vi "DFD NStage MRate Filtering (Array).vi"(6 "zero phase? (T)":bool=TRUE, 7 "init? (F)":bool, 8 "error in (no error)":errorcluster, 10 "multirate filters":T1[](array[typedef]) {"mMRate_SumWl" min=1 max=32 step=1; "mMRate_InputIwl" min=1 max=32 step=1; "mMRate_GainWl" min=1 max=32 step=1; "mMRate_OutputWl" min=1 max=32 step=1; "mMRate_InputWl" min=1 max=32 step=1; "mMRate_CoefWl" min=1 max=32 step=1; "mMRate_Mode" items=["Default"=-1, "No Rate Change"=0, "Interpolation"=1, "Decimation"=2, "Interpolated"=3, "Rational"=4]}, 11 "signal in":dbl[](array[numeric])) -> (0 "error out":errorcluster, 3 "signal out":dbl[](array[numeric]))   [LabVIEW 2017, in "NI_DigFilterLicensed.lvlib"]
doc: "Filters a signal continuously with a multistage multirate filter. Wire data to the <B>signal in</B> input to determine the polymorphic instance to use or manually select the instance."
uses:
  <vilib>/addons/Digital Filter Design/NI_DigFilterLicensed.lvlib
  <vilib>/addons/Digital Filter Design/_Objects.llb/DFD Multirate Filter Obj.ctl
  <vilib>/addons/Digital Filter Design/_Objects.llb/DFD Multirate Mode.ctl
  <vilib>/addons/Digital Filter Design/_Objects.llb/DFD Coef Norm Type.ctl
  <vilib>/addons/Digital Filter Design/_Objects.llb/DFD Round-off Mode.ctl
  <vilib>/addons/Digital Filter Design/_Objects.llb/DFD FXP MRate Multiply Mode.ctl
  <vilib>/addons/Digital Filter Design/NI_DigFilter_Process.lvlib
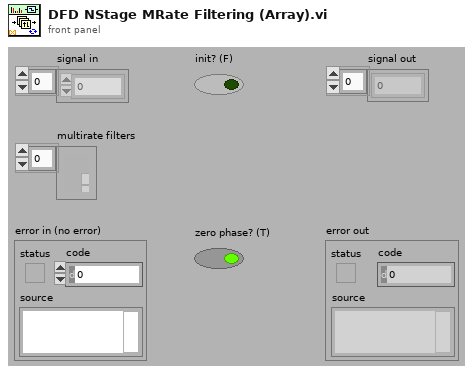
[diagram p1: front panel]
types:
  T1 = typedef "NI_DigFilterLicensed.lvlib/DFD Multirate Filter Obj.ctl" = cluster{"mMRate_Structure":enum16{"CIC", "FIR", "IIR", "Lattice"}, "mMRate_Mode":T2, "mMRate_Factor":i32, "mMRate_FIRParams":cluster{"mMRate_FIR_H":dbl[], "mMRate_FIR_IsNyquist?":bool, "mMRate_FIR_IsSymmetric?":bool}, "mMRate_CICParams":cluster{"mMRate_CIC_#Stage":i32, "mMRate_CIC_Lag":i32, "mMRate_CIC_Type":enum16{"Lowpass", "Highpass"}}, "mMRate_Order":i32, "mMRate_Version":string, "mMRate_Comments":string, "mMRate_RationalFactor":cluster{"mMRate_L":i32, "mMRate_M":i32}, "mMRate_Fs":dbl, "mMRate_Quantized?":bool, "mMRate_QFilterGain":dbl, "mMRate_CoefWl":i16, "mMRate_Scaling":cluster{"mMRate_ScaleByPowerOf2?":bool, "mMRate_ScaleType":T3}, "mMRate_InputWl":i16, "mMRate_OutputWl":i16, "mMRate_OutputMode":T4, "mMRate_MultMode":T5, "mMRate_BitPruning":bool, "mMRate_GainWl":i16, "mMRate_OutputFwl":i16, "mMRate_SumIwl":i16, "mMRate_InputIwl ":i16, "mMRate_SumWl":i16, "mMRate_CoefIwl":i16}
  T2 = typedef "NI_DigFilterLicensed.lvlib/DFD Multirate Mode.ctl" = i16
  T3 = typedef "NI_DigFilterLicensed.lvlib/DFD Coef Norm Type.ctl" = enum16{"No Norm", "Time Domain 1-Norm", "Time Domain 2-Norm", "Time Domain Inf-Norm"}
  T4 = typedef "NI_DigFilterLicensed.lvlib/DFD Round-off Mode.ctl" = enum16{"Nearest", "Truncation"}
  T5 = typedef "NI_DigFilterLicensed.lvlib/DFD FXP MRate Multiply Mode.ctl" = enum16{"Truncated", "Full"}
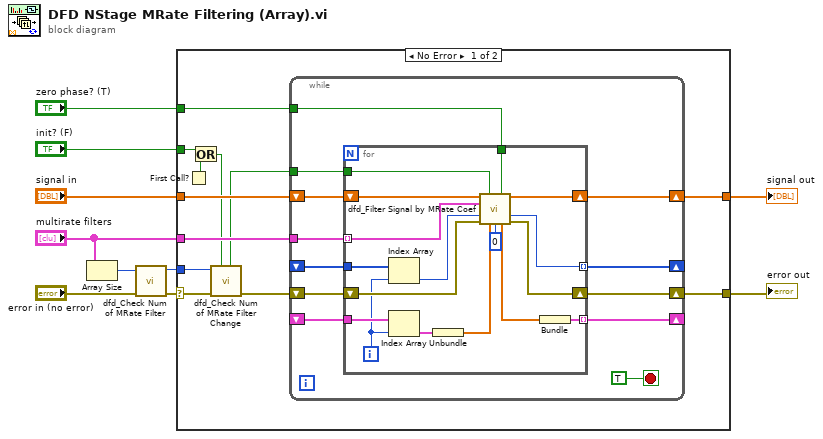
[diagram p0: block diagram]
diagram:
  n1 = Array Size(array="multirate filters") -> (size(s)=w3:i32)
  n2 = call <vilib>:"dfd_Check Num of MRate Filter.vi"("error in (no error)"="error in (no error)", "#MRate in"=w3) -> ("error out"=w4:errorcluster, "#MRate out"=w1:i32)  [unwired: 8 out]
  n3 = case shown="No Error" w4 {
    selector: w4 -> [w15 w52]
    tunnel: [w22 w52] -> w10
    tunnel: "multirate filters" -> [w16 _]
    tunnel: "signal in" -> [w17 _]
    tunnel: [w20 _] -> w8
    tunnel: "zero phase? (T)" -> [w21 _]
    tunnel: "init? (F)" -> [w18 _]
    tunnel: w1 -> [w11 _]
    frame No Error {
      n4 = First Call?() -> (First Call?: T/F=w19:bool)
      n5 = Or(x=w18, y=w19) -> (x .or. y?=w13:bool)
      n6 = call <vilib>:"dfd_Check Num of MRate Filter Change.vi"("init in"=w13, "error in (no error)"=w15, "#MRate in"=w11) -> ("error out"=w14:errorcluster, "init out"=w12:bool)  [unwired: 7 out]
      n7 = while {
        tunnel: w16 -> [w34]
        shift-right: [w32] -> _
        shift-left: _ -> [w26]
        tunnel: w12 -> [w27]
        shift-right: [w30] -> _
        shift-left: _ -> [w24]
        tunnel: w21 -> [w23]
        shift-right: [w25] -> w22
        shift-left: w14 -> [w31]
        shift-right: [w28] -> w20
        shift-left: w17 -> [w29]
        stop <- TRUE stop-if-true
        n8 = for {
          tunnel: w34 -> [w47] mode=indexing
          tunnel: [w51] -> w32 mode=indexing
          tunnel: w26 -> [w50]
          tunnel: [w46] -> w30 mode=indexing
          tunnel: w27 -> [w35]
          tunnel: w23 -> [w45]
          shift-right: [w44] -> w28
          shift-left: w29 -> [w48]
          shift-right: [w36] -> w25
          shift-left: w31 -> [w40]
          tunnel: w24 -> [w38]
          i -> [w39]
          n9 = Index Array(array=w38, index=w39) -> (element=w37:i32)
          n10 = Index Array(array=w50, index=w39) -> (element=w49:cluster{"state out":dbl[]})
          n11 = Unbundle(w49) -> ("state out"=w41:dbl[])
          n12 = call <vilib>:"dfd_Filter Signal by MRate Coef.vi"("signal in"=w48, "initH?"=w35, "zeroPhaseH?"=w45, "multirate filter"=w47, "skipPoint In"=w37, "error in (no error)"=w40, "state in"=w41, "outputPhase"=0) -> ("signal out"=w44:dbl[], "skipPoint Out"=w46:i32, "state out"=w43:dbl[], "error out"=w36:errorcluster)  [unwired: 4 out]
          n13 = Bundle("state out"=w43) -> (w51:cluster{"state out":dbl[]})  [unwired: 1 in]
        }
      }
    }
    frame Error {
    }
  }
  "error out" <- w10
  "signal out" <- w8
